vi "Conditional Not.vi"(9 "Input":bool, 10 "Not?":bool) -> (1 "Output":bool)   [LabVIEW 2014]
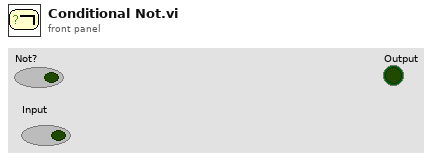
[diagram p1: front panel]
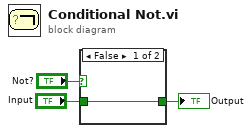
[diagram p0: block diagram]
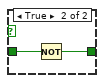
[diagram p2: hidden frame]
diagram:
  n1 = case shown="False" "Not?" {
    tunnel: "Input" -> [w4 w6]
    tunnel: [w4 w5] -> w1
    frame False {
    }
    frame True {
      n2 = Not(x=w6) -> (.not. x?=w5:bool)
    }
  }
  "Output" <- w1
